vi "Step.vi"(1 "Control in":T1={"queue"=refnum, "error"={"status"=FALSE, "code"=0, "source"=""}, "Step"={"Name"="", "Timeout"=0.0}, "Algorythm"=[{"Name"="Init", "Timeout"=0.0}]}) -> (9 "Init?":bool, 13 "Name":string, 15 "Control out":T1={"queue"=refnum, "error"={"status"=FALSE, "code"=0, "source"=""}, "Step"={"Name"="", "Timeout"=0.0}, "Algorythm"=[{"Name"="Init", "Timeout"=0.0}]})   [LabVIEW 2023, in "SFC.lvlib"]
uses:
  SFC.lvlib
  TypeDef/Control TypeDef.ctl
  TypeDef/Step TypeDef.ctl
  6bfdc3b9-b4f2-4c01-9504-a9ba17223ff4.vi
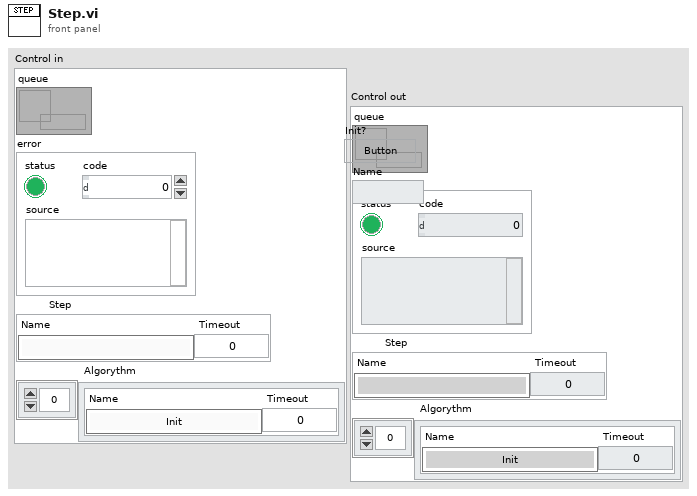
[diagram p1: front panel]
types:
  T1 = typedef "SFC.lvlib/Control TypeDef.ctl" = cluster{"queue":refnum<queue>, "error":errorcluster, "Step":T2, "Algorythm":T2[]}
  T2 = typedef "SFC.lvlib/Step TypeDef.ctl" = cluster{"Name":string, "Timeout":dbl}
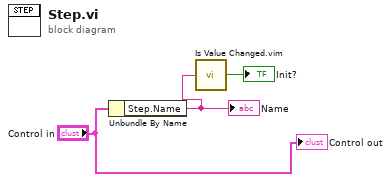
[diagram p0: block diagram]
diagram:
  n1 = Unbundle By Name("Control in") -> ("Step.Name"=w3:string)
  "Name" <- w3
  n2 = call "Is Value Changed.vim"("value"=w3) -> ("changed or first call?"=→"Init?":bool)
  "Control out" <- "Control in"
